vi "MODBUS RTU Receive Message.vi"(6 "Receive Message Type (0: By The Number Of Bytes)":u16(ring) items=["By The Number Of Bytes", "Copy Of The Sent Message"], 8 "error in (no error)":errorcluster, 9 "Sent Command (0)":u8, 10 "Length Of Sent MSG (0)":u8, 11 "VISA session":refnum<visa-resource-name>) -> (0 "error out":errorcluster, 1 "Read Buffer":u8[](array[numeric]), 3 "dup VISA session":refnum<visa-resource-name>)   [LabVIEW 2017]
doc: "VI - receive MODBUS RTU frame described by <B>Sent Command</B> control <LengthOfSentMSG> control (set out by MODBUS RTU Send Message.vi) and\nby selection <B>Receive Message Type</B>.\n\nThis VI is without message content decoding.\nSeparate usefull data message\nfrom the rest of the data frame and put it to the <B>read Buffer</B>.\nThe selector decode the frame by type of reading - \n\nAnswers can have 2 types:\n\n1. in answer frame is copy of the frame - is need to initialize on the input - <B>LengthOfSentMSG</B> and <B>Sent Command</B>, for right decoding\n\n2. answer frame consists information about length of main message in frame - The frame is divided automatically\n\n\nDescribed errors:\nBFFC09F1 - Bad in back protocol in Write Operation. Transmit Error.\nBFFC09F2 - Bad Received Message CRC\nBFFC09F3 - After WRITE: Error Statement, Error CRC\nBFFC09F4 - After WRITE: Register don't exist or is only for reading\nBFFC09F5 - After WRITE: data out of borders"
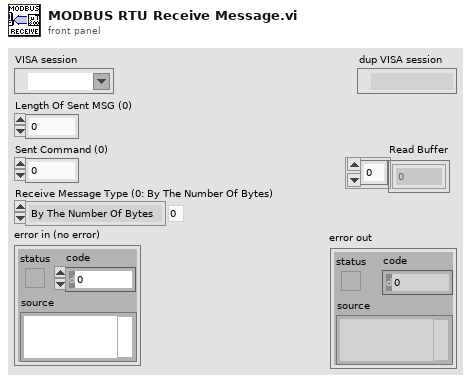
[diagram p1: front panel]
types:
  T1 = cluster{"unsigned byte array[0]":u8, "unsigned byte array[1]":u8}
  T2 = cluster{"status":bool, "code":i32, "VI Name":string}
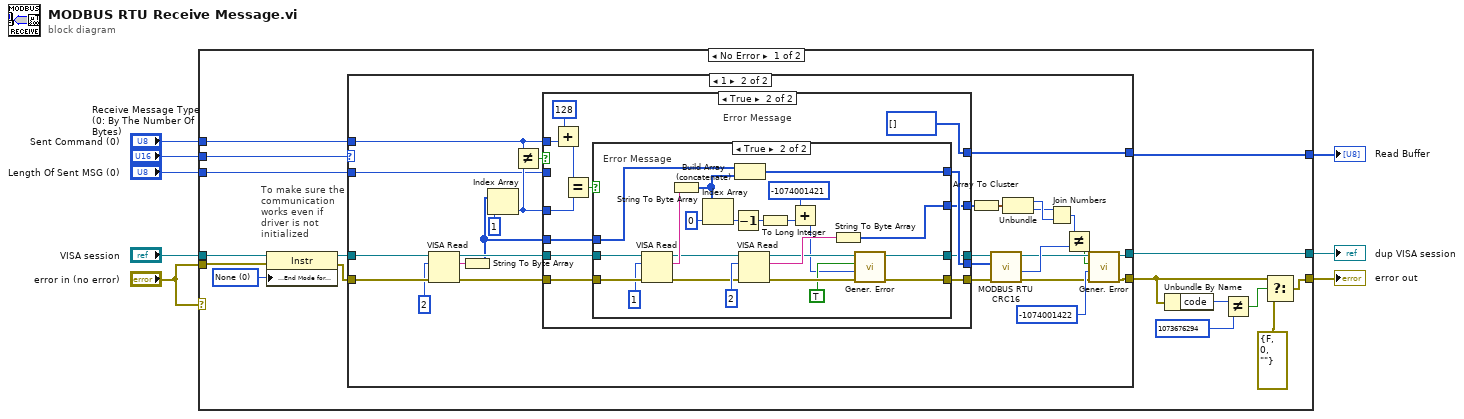
[diagram p0: block diagram]
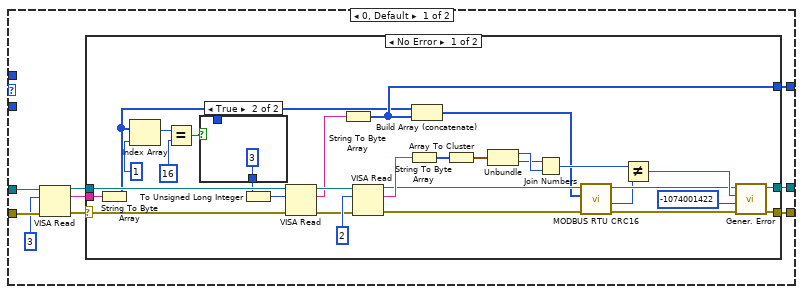
[diagram p2: hidden frame]
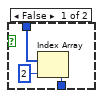
[diagram p3: hidden frame]
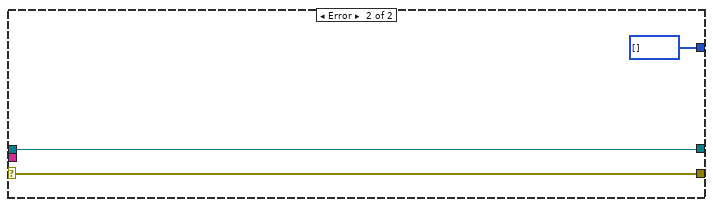
[diagram p4: hidden frame]
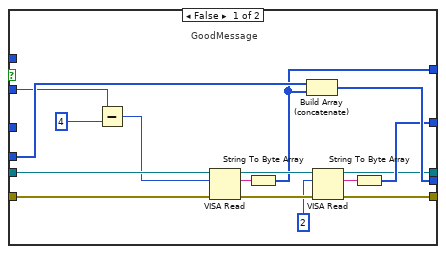
[diagram p5: hidden frame]
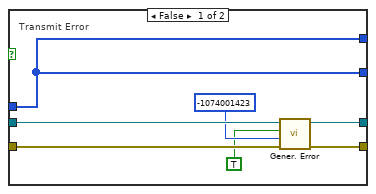
[diagram p6: hidden frame]
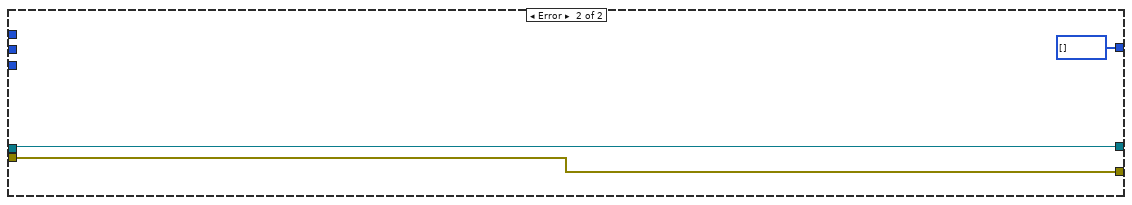
[diagram p7: hidden frame]
diagram:
  n1 = case shown="No Error" "error in (no error)" {
    tunnel: "error in (no error)" -> [w11 w160]
    tunnel: "Receive Message Type (0: By The Number Of Bytes)" -> [w24 _]
    tunnel: "VISA session" -> [w13 w159]
    tunnel: "Length Of Sent MSG (0)" -> [w23 _]
    tunnel: "Sent Command (0)" -> [w22 _]
    tunnel: [w21 u8[] [] ("unsigned byte array")] -> w4
    tunnel: [w15 w159] -> w2
    tunnel: [w14 w160] -> w1
    frame No Error {
      w9 = u16 0 items=["None", "LastBit", "TermChar"] ("Serial Settings:Serial End Mode for Reads")
      # "To make sure the\ncommunication \nworks even if\ndriver is not \ninitialized"
      n2 = property class="Instr"(reference=w13, error in=w11, "Serial Settings:End Mode for Reads"=w9) -> (reference out=w12:refnum<visa-resource-name>, error out=w10:errorcluster)
      n3 = case shown="1" w24 {
        tunnel: [w28 w76] -> w20
        tunnel: w10 -> [w33 w98]
        tunnel: w12 -> [w31 w99]
        tunnel: [w26 w77] -> w15
        tunnel: [w25 w86] -> w21
        tunnel: w23 -> [_ w82]
        tunnel: w22 -> [_ w88]
        frame 0, Default {
          n4 = VISA Read(VISA resource name=w31, byte count=u32 3 ("byte count (0)"), error in (no error)=w33) -> (VISA resource name out=w27:refnum<visa-resource-name>, read buffer=w30:string, error out=w29:errorcluster)  [unwired: 1 out]
          n5 = case shown="No Error" w29 {
            selector: w29 -> [w63 w71]
            tunnel: w30 -> [w64 _]
            tunnel: [w42 w71] -> w28
            tunnel: w27 -> [w62 w70]
            tunnel: [w52 u8[] [] ("unsigned byte array")] -> w25
            tunnel: [w43 w70] -> w26
            frame No Error {
              n6 = String To Byte Array(string=w64) -> (unsigned byte array=w45:u8[])
              n7 = Index Array(array=w45, index=1) -> (element=w47:u8)
              n8 = Equal?(x=w47, y=u8 16 ("x")) -> (x = y?=w46:bool)
              n9 = case shown="True" w46 {
                tunnel: [w66 u8 3] -> w44
                tunnel: w45 -> [w65 _]
                frame False {
                  n10 = Index Array(array=w65, index=2) -> (element=w66:u8)
                }
                frame True {
                }
              }
              n11 = To Unsigned Long Integer(number=w44) -> (unsigned 32bit integer=w50:u32)
              n12 = VISA Read(VISA resource name=w62, byte count=w50, error in (no error)=w63) -> (VISA resource name out=w59:refnum<visa-resource-name>, read buffer=w57:string, error out=w58:errorcluster)  [unwired: 1 out]
              n13 = String To Byte Array(string=w57) -> (unsigned byte array=w52:u8[])
              n14 = VISA Read(VISA resource name=w59, byte count=u32 2 ("byte count (0)"), error in (no error)=w58) -> (VISA resource name out=w36:refnum<visa-resource-name>, read buffer=w61:string, error out=w39:errorcluster)  [unwired: 1 out]
              n15 = String To Byte Array(string=w61) -> (unsigned byte array=w56:u8[])
              n16 = Build Array (concatenate)(w45, w52) -> (w35:u8[])
              n17 = Array To Cluster(array=w56) -> (cluster=w55:T1)
              n18 = Unbundle(w55) -> ("unsigned byte array[0]"=w54:u8, "unsigned byte array[1]"=w53:u8)
              n19 = Join Numbers(hi=w53, lo=w54) -> ((hi.lo)=w51:u16)
              n20 = call "MODBUS RTU CRC16.vi"("error in (no error)"=w39, "Message (empty array)"=w35, "VISA session"=w36) -> ("error out"=w38:errorcluster, "CRC"=w34:u16, "dup VISA session"=w37:refnum<visa-resource-name>)  [unwired: 5 in, 1 out]
              n21 = Not Equal?(x=w51, y=w34) -> (x != y?=w40:bool)
              n22 = call "Gener. Error.vi"("error in (no error)"=w38, "Code (0)"=-1074001422, "Status (F: Off)"=w40, "VISA session"=w37) -> ("error out"=w42:errorcluster, "dup VISA session"=w43:refnum<visa-resource-name>)  [unwired: 6 in]
            }
            frame Error {
            }
          }
        }
        frame 1 {
          n23 = VISA Read(VISA resource name=w99, byte count=u32 2 ("byte count (0)"), error in (no error)=w98) -> (VISA resource name out=w97:refnum<visa-resource-name>, read buffer=w83:string, error out=w92:errorcluster)  [unwired: 1 out]
          n24 = String To Byte Array(string=w83) -> (unsigned byte array=w87:u8[])
          n25 = Index Array(array=w87, index=1) -> (element=w89:u8)
          n26 = Not Equal?(x=w88, y=w89) -> (x != y?=w90:bool)
          n27 = case shown="True" w90 {
            tunnel: w97 -> [w114 w128]
            tunnel: [w105 w119] -> w93
            tunnel: [w111 w121] -> w81
            tunnel: w92 -> [w115 w127]
            tunnel: w89 -> [_ w126]
            tunnel: w88 -> [_ w117]
            tunnel: [w107 w123] -> w79
            tunnel: w87 -> [w113 w122]
            tunnel: [w104 w120] -> w80
            tunnel: [w103 u8[] [] ("unsigned byte array")] -> w86
            tunnel: w82 -> [w102 _]
            frame False {
              # "GoodMessage"
              n28 = Subtract(x=w102, y=u8 4) -> (x-y=w101:u8)
              n29 = VISA Read(VISA resource name=w114, byte count=w101, error in (no error)=w115) -> (VISA resource name out=w109:refnum<visa-resource-name>, read buffer=w112:string, error out=w110:errorcluster)  [unwired: 1 out]
              n30 = String To Byte Array(string=w112) -> (unsigned byte array=w103:u8[])
              n31 = Build Array (concatenate)(w113, w103) -> (w111:u8[])
              n32 = VISA Read(VISA resource name=w109, byte count=u32 2 ("byte count (0)"), error in (no error)=w110) -> (VISA resource name out=w104:refnum<visa-resource-name>, read buffer=w106:string, error out=w107:errorcluster)  [unwired: 1 out]
              n33 = String To Byte Array(string=w106) -> (unsigned byte array=w105:u8[])
            }
            frame True {
              # "Error Message"
              n34 = Add(x=u8 128 ("y"), y=w117) -> (x+y=w125:u8)
              n35 = Equal?(x=w125, y=w126) -> (x = y?=w124:bool)
              n36 = case shown="True" w124 {
                tunnel: w128 -> [w133 w158]
                tunnel: w127 -> [w132 w157]
                tunnel: [w131 w140] -> w123
                tunnel: w122 -> [w135 w148]
                tunnel: [w135 w147] -> w121
                tunnel: [w134 w141] -> w120
                tunnel: [w135 w144] -> w119
                frame False {
                  # "Transmit Error"
                  n37 = call "Gener. Error.vi"("error in (no error)"=w132, "Code (0)"=-1074001423, "Status (F: Off)"=TRUE ("status"), "VISA session"=w133) -> ("error out"=w131:errorcluster, "dup VISA session"=w134:refnum<visa-resource-name>)  [unwired: 6 in]
                }
                frame True {
                  # "Error Message"
                  n38 = VISA Read(VISA resource name=w158, byte count=u32 1 ("byte count (0)"), error in (no error)=w157) -> (VISA resource name out=w143:refnum<visa-resource-name>, read buffer=w155:string, error out=w142:errorcluster)  [unwired: 1 out]
                  n39 = String To Byte Array(string=w155) -> (unsigned byte array=w154:u8[])
                  n40 = Index Array(array=w154, index=0) -> (element=w152:u8)
                  n41 = Decrement(x=w152) -> (x-1=w150:u8)
                  n42 = Build Array (concatenate)(w148, w154) -> (w147:u8[])
                  n43 = VISA Read(VISA resource name=w143, byte count=u32 2 ("byte count (0)"), error in (no error)=w142) -> (VISA resource name out=w139:refnum<visa-resource-name>, read buffer=w145:string, error out=w138:errorcluster)  [unwired: 1 out]
                  n44 = To Long Integer(number=w150) -> (32bit integer=w149:i32)
                  n45 = Add(x=-1074001421, y=w149) -> (x+y=w136:i32)
                  n46 = String To Byte Array(string=w145) -> (unsigned byte array=w144:u8[])
                  n47 = call "Gener. Error.vi"("error in (no error)"=w138, "Code (0)"=w136, "Status (F: Off)"=TRUE ("status"), "VISA session"=w139) -> ("error out"=w140:errorcluster, "dup VISA session"=w141:refnum<visa-resource-name>)  [unwired: 6 in]
                }
              }
            }
          }
          n48 = Array To Cluster(array=w93) -> (cluster=w96:T1)
          n49 = call "MODBUS RTU CRC16.vi"("error in (no error)"=w79, "Message (empty array)"=w81, "VISA session"=w80) -> ("error out"=w74:errorcluster, "CRC"=w78:u16, "dup VISA session"=w73:refnum<visa-resource-name>)  [unwired: 5 in, 1 out]
          n50 = Unbundle(w96) -> ("unsigned byte array[0]"=w95:u8, "unsigned byte array[1]"=w94:u8)
          n51 = Join Numbers(hi=w94, lo=w95) -> ((hi.lo)=w85:u16)
          n52 = Not Equal?(x=w85, y=w78) -> (x != y?=w72:bool)
          n53 = call "Gener. Error.vi"("error in (no error)"=w74, "Code (0)"=-1074001422, "Status (F: Off)"=w72, "VISA session"=w73) -> ("error out"=w76:errorcluster, "dup VISA session"=w77:refnum<visa-resource-name>)  [unwired: 6 in]
        }
      }
      n54 = Unbundle By Name(w20) -> ("code"=w19:i32)
      n55 = Not Equal?(x=w19, y=1073676294) -> (x != y?=w17:bool)
      n56 = Select(t=w20, s=w17, f=cluster{bool, i32, "VI Name":string} {FALSE, 0, "VI Name"=""}) -> (s? t:f=w14:T2)
    }
    frame Error {
    }
  }
  "error out" <- w1
  "dup VISA session" <- w2
  "Read Buffer" <- w4
